vi "gds_rx_top.vi"(0 "Modulation Parameters":T4={"RX Parameters"={"Sampling Rate"=1000000.0, "RX Oversample Factor"=2}, "Shared Parameters"={"Packet Length"=500, "Preamble Length"=20, "modulation type"=enum."OOK", "FSK deviation (Hz)"=625.0, "Filter Parameters"={"modulation type"=enum."ASK", "pulse shaping filter (none)"=enum."none", "filter length (symbols)"=8, "filter parameter"=0.5}}}, 1 "HW parameters":T5={"Device IP Address"="192.168.10.26", "Active Antenna"="RX2", "Carrier Frequency (Hz)"=433000000.0, "Gain (dB)"=20.0, "Trigger Level"=0.01, "Bandwidth (Hz)"=40000000.0, "Reference Position (%)"=10.0, "Capture Time (s)"=0.0001, "Simulate"=FALSE} {"Capture Time (s)" format="%.2p"; "Bandwidth (Hz)" format="%.2p"; "Trigger Level" format="%#.3p"; "Gain (dB)" format="%.2f"; "Carrier Frequency (Hz)" format="%.2p"}, 2 "Received Bit Sequence":i8[](array[numeric]) caption="Received Key Bit Sequence", 3 "Received IQ\nwaveform":cluster{"t0":dbl, "dt":dbl, "Y":cdb[]} {"Y" format="%.2g"; "dt" format="%.2g"; "t0" format="%.2g"}, 4 "stop":bool, 5 "error in":errorcluster, 6 "# of Receive Iterations":u16=1) -> (7 "coerced carrier frequency (Hz)":dbl format="%#_6p", 10 "I":waveform(dbl)(graph), 11 "coerced bandwidth":dbl, 12 "Q":waveform(dbl)(graph), 13 "coerced gain (dB)":dbl format="%#_6f", 14 "recovered complex waveform":T2 {"Y" format="%.3f"; "dt" format="%^.2e"; "t0" format="%.4f"}, 15 "bit-error rate":dbl, 17 "average \nbit-error rate":dbl, 18 "key bit sequence":i8[](array[numeric]), 19 "error out":errorcluster)   [LabVIEW 2012]
uses:
  EE 497/LABS/SDR/control_type_defs.llb/rx_hw params.ctl
  <vilib>/addons/Modulation/Analog/controls/Complex Data Waveform.ctl
  <vilib>/Analysis/baseanly.llb/Mean (DBL).vi
  <vilib>/addons/Modulation/niAMT.lvlib
  <vilib>/Analysis/NI_AALBase.lvlib
panel:
  out "Measurements":T1 caption="measurements" {"FSK error (Hz)" format="%.2f"; "deviation error (Hz)" format="%.2f"; "frequency drift (Hz)" format="%.2f"; "frequency offset (Hz)" format="%.2f"}
  out "Packet Detected":bool
  in  "Configurations":T3(tab)
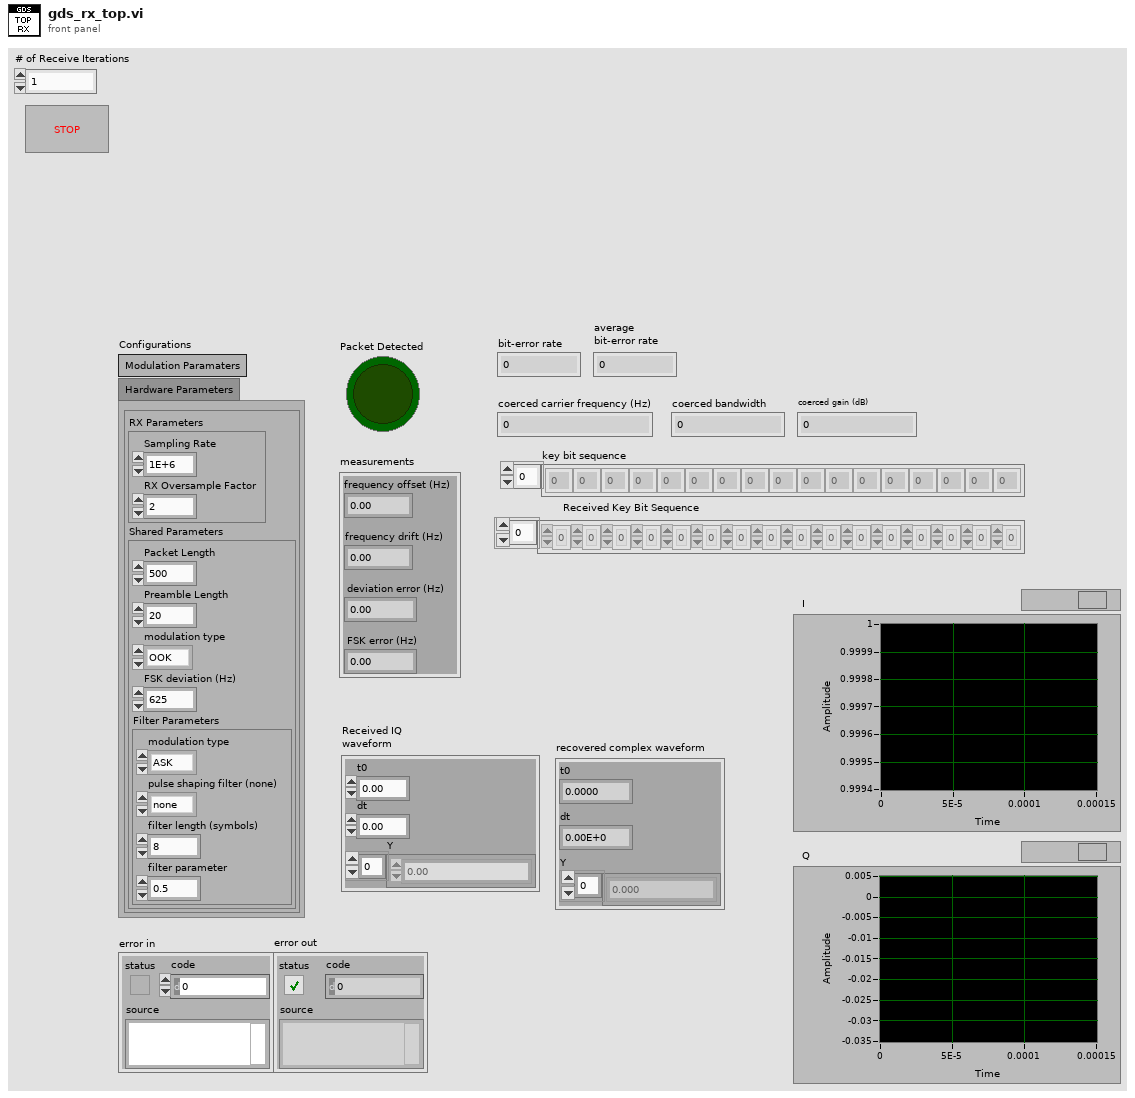
[diagram p1: front panel]
types:
  T1 = cluster{"frequency offset (Hz)":dbl, "frequency drift (Hz)":dbl, "deviation error (Hz)":dbl, "FSK error (Hz)":dbl}
  T2 = typedef "niAMT.lvlib/Complex Data Waveform.ctl" = cluster{"t0":dbl, "dt":dbl, "Y":cdb[]}
  T3 = enum32{"Modulation Paramaters", "Hardware Parameters"}
  T4 = cluster{"RX Parameters":cluster{"Sampling Rate":dbl, "RX Oversample Factor":i32}, "Shared Parameters":cluster{"Packet Length":i32, "Preamble Length":i32, "modulation type":enum16{"OOK", "FSK", "PSK", "QAM", "MSK", "PAM", "ASK", "CPM"}, "FSK deviation (Hz)":dbl, "Filter Parameters":cluster{"modulation type":enum16{"FSK", "PSK", "QAM", "MSK", "PAM", "ASK", "CPM"}, "pulse shaping filter (none)":enum16{"none", "Raised Cosine", "Root Raised Cos", "Gaussian"}, "filter length (symbols)":i32, "filter parameter":dbl}}}
  T5 = typedef "rx_hw params.ctl" = cluster{"Device IP Address":refnum<k15>, "Active Antenna":string, "Carrier Frequency (Hz)":dbl, "Gain (dB)":dbl, "Trigger Level":dbl, "Bandwidth (Hz)":dbl, "Reference Position (%)":dbl, "Capture Time (s)":dbl, "Simulate":bool}
  T6 = cluster{"Sampling Rate":dbl, "RX Oversample Factor":i32}
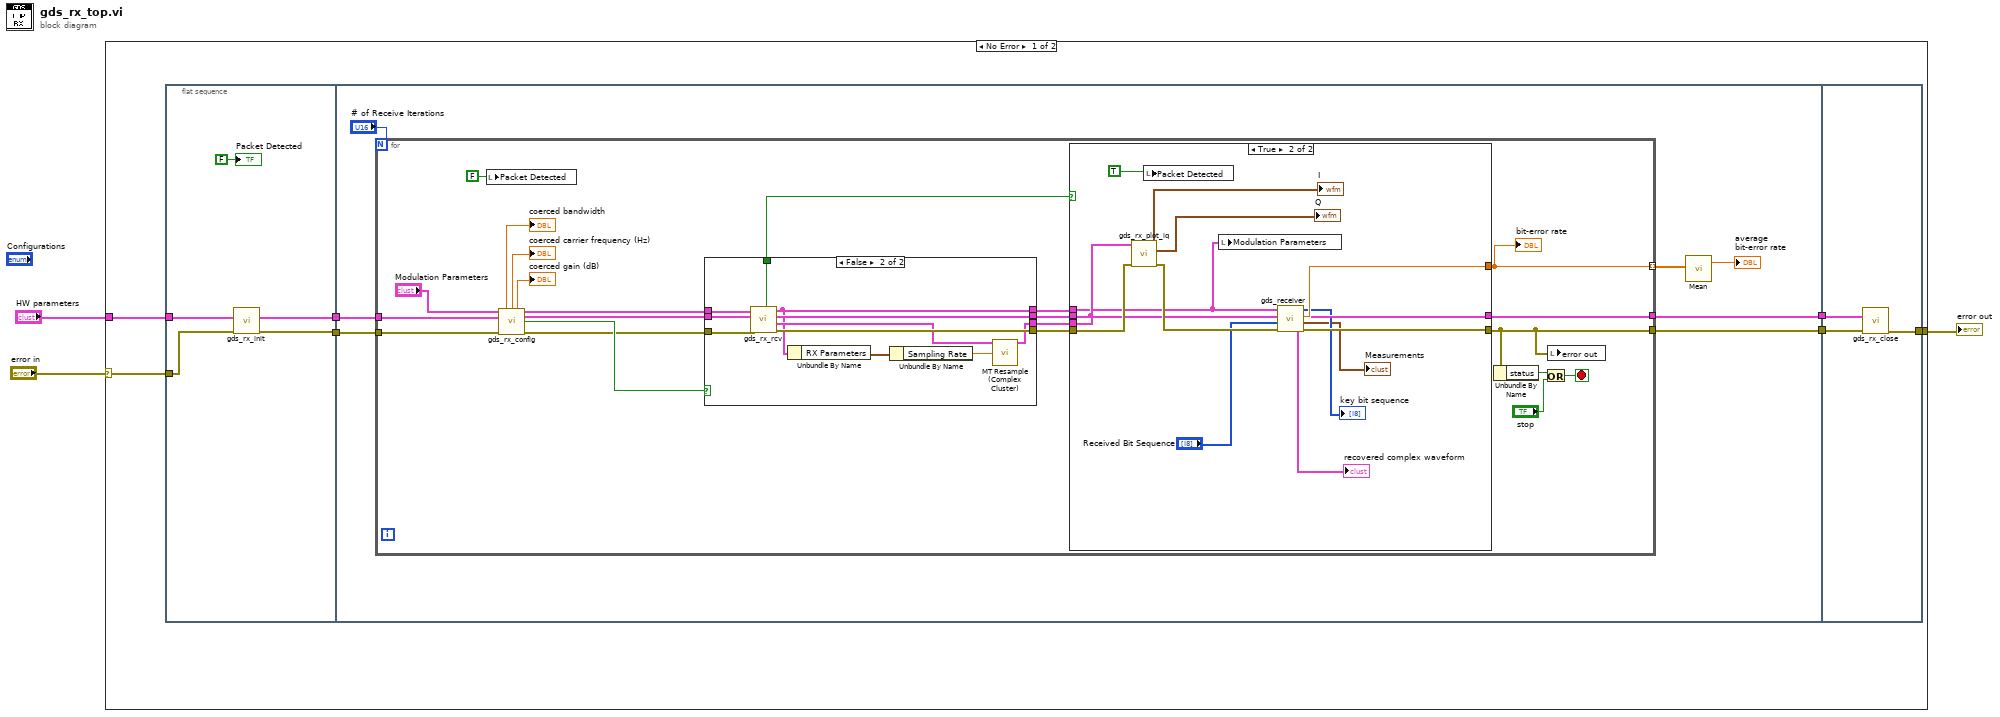
[diagram p0: block diagram]
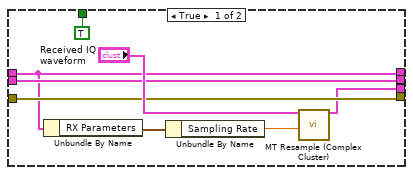
[diagram p3: hidden frame]
diagram:
  n1 = case shown="No Error" "error in" {
    selector: "error in" -> [w9 w83]
    tunnel: "HW parameters" -> [w10 _]
    tunnel: [w6 w83] -> w1
    frame No Error {
      n2 = flat-sequence {
        tunnel: w10 -> [w14]
        tunnel: w9 -> [w13]
        tunnel: [w12] -> w8
        tunnel: [w11] -> w5
        tunnel: w8 -> [w21]
        tunnel: [w20] -> w7
        tunnel: w5 -> [w17]
        tunnel: [w16] -> w4
        tunnel: w7 -> [w82]
        tunnel: [w81] -> w6
        tunnel: w4 -> [w80]
        frame #0 {
          n3 = call "gds_rx_init.vi"("error in (no error)"=w13, "HW parameters In"=w14) -> ("error out"=w12:errorcluster, "HW parameters Out"=w11:T5)  [unwired: 7 in, 1 out]
          "Packet Detected" <- FALSE ("Packet Detected")
        }
        frame #1 {
          n4 = for {
            N: "# of Receive Iterations" -> [_]
            tunnel: w21 -> [w43]
            tunnel: [w29] -> w20
            tunnel: [w28] -> w19 mode=indexing
            tunnel: w17 -> [w27]
            tunnel: [w23] -> w16
            stop <- w30 stop-if-true
            n5 = local write "Packet Detected"(FALSE ("Packet Detected")) -> ()
            n6 = call "gds_rx_config.vi"("Modulation Parameters"="Modulation Parameters", "HW parameters In"=w27, "error in (no error)"=w43) -> ("coerced bandwidth"=→"coerced bandwidth":dbl, "coerced carrier frequency (Hz)"=→"coerced carrier frequency (Hz)":dbl, "coerced gain (dB)"=→"coerced gain (dB)":dbl, "Modulation Parameters Out"=w25:T4, "HW parameters Out"=w24:T5, "Simulate"=w39:bool, "error out"=w38:errorcluster)  [unwired: 6 in]
            n7 = case shown="False" w39 {
              tunnel: w38 -> [w66 w79]
              tunnel: [w66 w76] -> w33
              tunnel: [w65 w73] -> w34
              tunnel: [w61 w69] -> w36
              tunnel: [w62 w70] -> w35
              tunnel: [TRUE ("Packet Detected") w74] -> w37
              tunnel: w25 -> [w61 w72]
              tunnel: w24 -> [w62 w71]
              frame True {
                n8 = Unbundle By Name(w61) -> ("RX Parameters"=w64:T6)
                n9 = Unbundle By Name(w64) -> ("Sampling Rate"=w63:dbl)
                n10 = call <vilib>:"MT Resample (Complex Cluster).vi"("input complex waveform"="Received IQ\nwaveform", "desired sample rate (Hz)"=w63) -> ("output complex waveform"=w65:T2)  [unwired: 12 in, 1 out]
              }
              frame False {
                n11 = call "gds_rx_rcv.vi"("error in (no error)"=w79, "HW parameters In"=w71, "Modulation Parameters"=w72) -> ("error out"=w76:errorcluster, "Received IQ waveform"=w75:cluster{"t0":dbl, "dt":dbl, "Y":cdb[]}, "HW parameters Out"=w70:T5, "Modulation Parameters Out"=w69:T4, "Packet Detected"=w74:bool)  [unwired: 4 in]
                n12 = Unbundle By Name(w69) -> ("RX Parameters"=w78:T6)
                n13 = Unbundle By Name(w78) -> ("Sampling Rate"=w77:dbl)
                n14 = call <vilib>:"MT Resample (Complex Cluster).vi"("input complex waveform"=w75, "desired sample rate (Hz)"=w77) -> ("output complex waveform"=w73:T2)  [unwired: 12 in, 1 out]
              }
            }
            n15 = case shown="True" w37 {
              tunnel: w36 -> [_ w53]
              tunnel: w35 -> [w45 w54]
              tunnel: w34 -> [_ w56]
              tunnel: w33 -> [w46 w58]
              tunnel: [w46 w59] -> w29
              tunnel: [_ w55] -> w28
              tunnel: [w45 w54] -> w23
              frame False {
              }
              frame True {
                n16 = call "gds_rx_plot_iq.vi"("error in"=w58, "Received IQ\nwaveform"=w56) -> ("error out"=w57:errorcluster, "Q component"=→"Q":waveform(dbl), "I component"=→"I":waveform(dbl))  [unwired: 7 in]
                n17 = local write "Packet Detected"(TRUE ("Packet Detected")) -> ()
                n18 = local write "Modulation Parameters"(w53) -> ()
                n19 = call "gds_receiver.vi"("error in (no error)"=w57, "Received Bit Sequence"="Received Bit Sequence", "Received Signal"=w56, "Modulation Parameters"=w53) -> ("error out"=w59:errorcluster, "Measurements"=→"Measurements":T1, "BER"=w55:dbl, "Key Bit Sequence"=→"key bit sequence":i8[], "recovered complex waveform"=→"recovered complex waveform":T2)  [unwired: 3 in]
              }
            }
            "bit-error rate" <- w28
            n20 = Unbundle By Name(w29) -> ("status"=w32:bool)
            n21 = Or(x=w32, y="stop") -> (x .or. y?=w30:bool)
            n22 = local write "error out"(w29) -> ()
          }
          n23 = call-poly <vilib>:"Mean.vi"("X"=w19) -> ("mean"=→"average \nbit-error rate":dbl)  [unwired: 1 out]
        }
        frame #2 {
          n24 = call "gds_rx_close.vi"("error in"=w82, "HW parameters"=w80) -> ("error out"=w81:errorcluster)  [unwired: 9 in]
        }
      }
    }
    frame Error {
    }
  }
  "error out" <- w1
